vi "WaitBallTrajSkill.vi"(8 "error in (no error)":errorcluster, 9 "Robot":refnum<class "Robot.lvclass">, 10 "Game":refnum<class "Game.lvclass">, 11 "WaitBallTrajSkill in":refnum<class "WaitBallTrajSkill.lvclass">) -> (0 "error out":errorcluster, 2 "robot out":refnum<class "Robot.lvclass">, 3 "WaitBallTrajSkill out":refnum<class "WaitBallTrajSkill.lvclass">)   [LabVIEW 2023, in "WaitBallTrajSkill.lvclass"]
uses:
  WaitBallTrajSkill.lvclass
  Game_class/Game.lvclass
  Robot_class/Robot.lvclass
  Object_class/Object.lvclass/Object.ctl
  Game_class/Game.lvclass/Game.ctl
  Ball_class/Ball.lvclass/Ball.ctl
  Robot_class/Robot.lvclass/Robot.ctl
  Game_class/Read BallRef.vi
  Game_class/Read Utilities.lvclass.vi
  Game_class/Read FieldRef.vi
  Object_class/Read x.vi
  Object_class/Read y.vi
  Ball_class/Read v_x.vi
  Ball_class/Read v_y.vi
  Robot_class/Write dest_x.vi
  Robot_class/Write dest_y.vi
  Robot_class/Write dest_orientation.vi
  Ball_class/Ball.lvclass
  Utilities_class/Utilities.lvclass
  Field_class/Field.lvclass
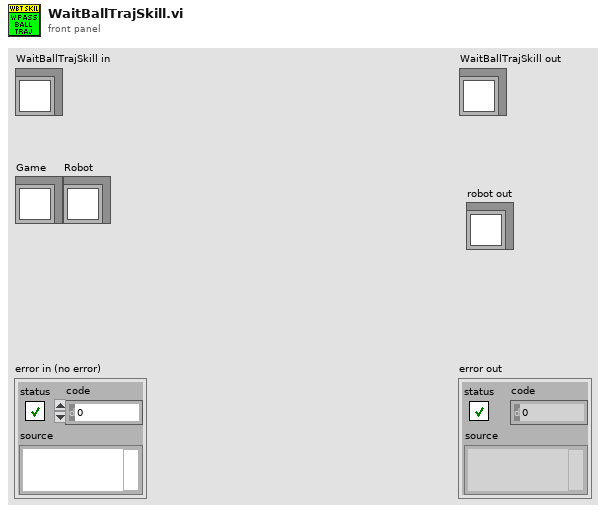
[diagram p1: front panel]
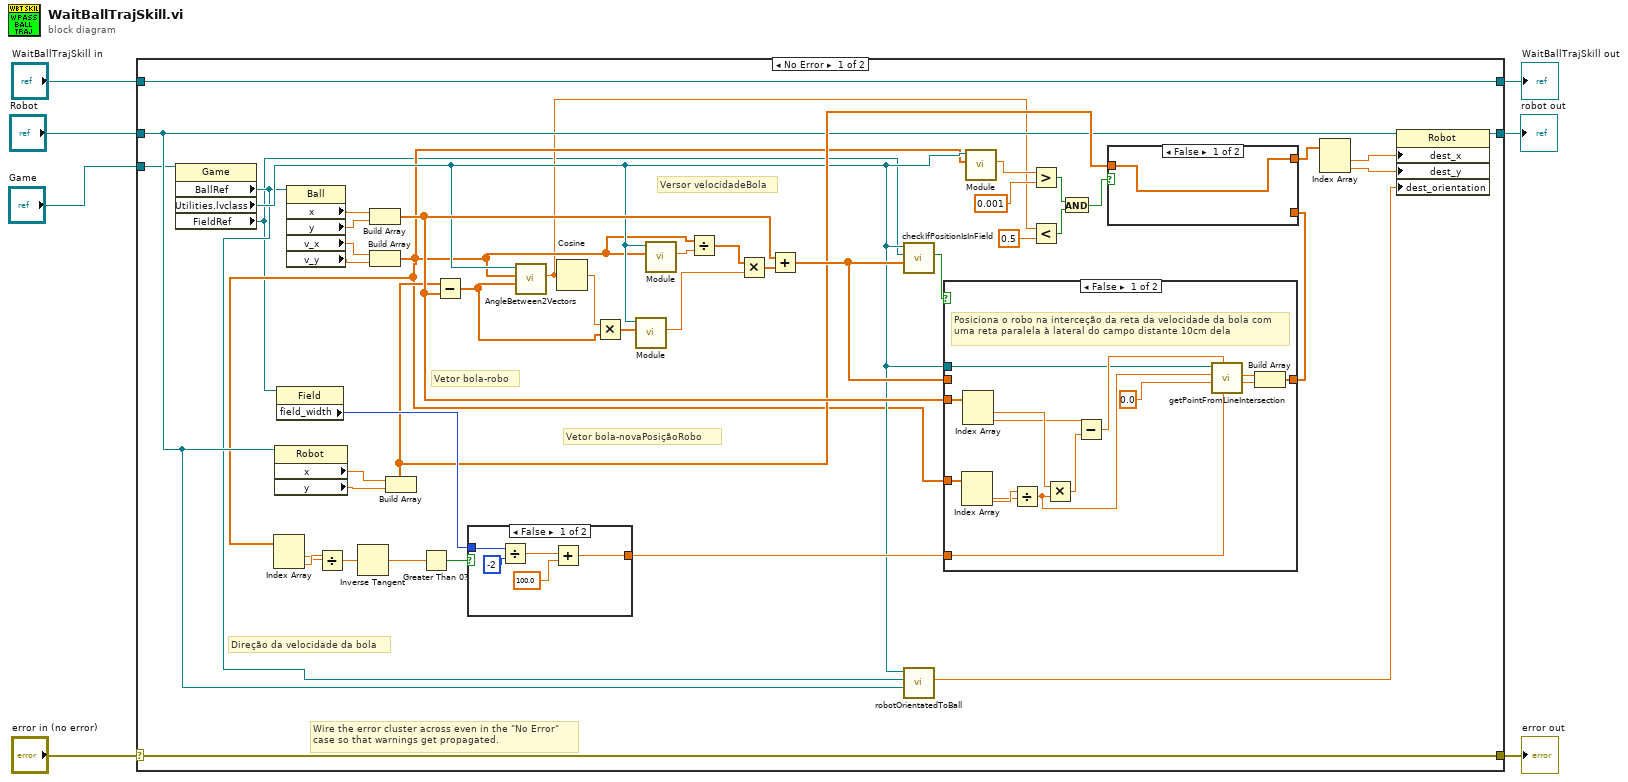
[diagram p0: block diagram]
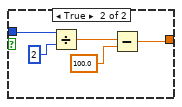
[diagram p3: hidden frame]
diagram:
  n1 = case shown="No Error" "error in (no error)" {
    selector: "error in (no error)" -> [w51 w82]
    tunnel: [w51 w82] -> w6
    tunnel: [w52 w81] -> w4
    tunnel: "WaitBallTrajSkill in" -> [w52 w81]
    tunnel: "Robot" -> [w23 _]
    tunnel: "Game" -> [w22 _]
    tunnel: [w50 _] -> w1
    frame No Error {
      # "Versor velocidadeBola"
      # "Direção da velocidade da bola"
      # "Vetor bola-novaPosiçãoRobo"
      # "Vetor bola-robo"
      # "Wire the error cluster across even in the \"No Error\"\ncase so that warnings get propagated."
      n2 = property class="Game"(reference=w22) -> ("BallRef"=w9:refnum<class "Ball.lvclass">, "Utilities.lvclass"=w20:refnum<class "Utilities.lvclass">, "FieldRef"=w8:refnum<class "Field.lvclass">)  [unwired: 1 in, 2 out]
      n3 = property class="Robot"(reference=w23) -> ("x"=w45:dbl, "y"=w44:dbl)  [unwired: 1 in, 2 out]
      n4 = property class="Field"(reference=w8) -> ("field_width"=w33:i32)  [unwired: 1 in, 2 out]
      n5 = property class="Ball"(reference=w9) -> ("x"=w49:dbl, "y"=w48:dbl, "v_x"=w46:dbl, "v_y"=w47:dbl)  [unwired: 1 in, 2 out]
      n6 = Build Array(w49, w48) -> (w31:dbl[])
      n7 = Build Array(w46, w47) -> (w18:dbl[])
      n8 = Index Array(array=w18) -> (element #1=w36:dbl, element #2=w37:dbl)  [unwired: 2 in]
      n9 = Divide(x=w37, y=w36) -> (x/y=w35:dbl)
      n10 = Inverse Tangent(1:w35) -> (0:w30:dbl)
      n11 = Build Array(w45, w44) -> (w25:dbl[])
      n12 = Greater Than 0?(x=w30) -> (x > 0?=w34:bool)
      n13 = Subtract(x=w25, y=w31) -> (x-y=w43:dbl[])
      n14 = case shown="False" w34 {
        tunnel: w33 -> [w58 w64]
        tunnel: [w57 w62] -> w32
        frame False {
          n15 = Divide(x=w58, y=-2) -> (x/y=w56:dbl)
          n16 = Add(x=w56, y=100.0) -> (x+y=w57:dbl)
        }
        frame True {
          n17 = Divide(x=w64, y=2) -> (x/y=w61:dbl)
          n18 = Subtract(x=w61, y=100.0) -> (x-y=w62:dbl)
        }
      }
      n19 = call "AngleBetween2Vectors.vi"("Array 1"=w43, "Array 2"=w18, "Utilities in"=w20) -> ("Numeric"=w10:dbl)  [unwired: 6 in, 2 out]
      n20 = Cosine(x=w10) -> (cos(x)=w42:dbl)
      n21 = Multiply(x=w42, y=w43) -> (x*y=w21:dbl[])
      n22 = call-dynamic "Module.vi"("2D vector"=w21, "Utilities in"=w20) -> ("Modulo"=w15:dbl)  [unwired: 7 in, 2 out]
      n23 = call-dynamic "Module.vi"("2D vector"=w18, "Utilities in"=w20) -> ("Modulo"=w19:dbl)  [unwired: 7 in, 2 out]
      n24 = Divide(x=w18, y=w19) -> (x/y=w16:dbl[])
      n25 = Multiply(x=w16, y=w15) -> (x*y=w17:dbl[])
      n26 = Add(x=w31, y=w17) -> (x+y=w40:dbl[])
      n27 = call "checkIfPositionIsInField.vi"("Position"=w40, "FieldRef"=w8, "Utilities in"=w20) -> ("Position Is In Field?"=w41:bool)  [unwired: 4 in, 4 out]
      n28 = call "robotOrientatedToBall.vi"("Robot"=w23, "BallRef"=w9, "Utilities in"=w20) -> ("Orientation"=w24:dbl)  [unwired: 6 in, 2 out]
      n29 = case shown="False" w41 {
        tunnel: w40 -> [_ w80]
        tunnel: [w77 w80] -> w29
        tunnel: w32 -> [w75 _]
        tunnel: w31 -> [w74 _]
        tunnel: w18 -> [w73 _]
        tunnel: w20 -> [w65 _]
        frame False {
          # "Posiciona o robo na interceção da reta da velocidade da bola com uma reta paralela à lateral do campo distante 10cm dela"
          n30 = Index Array(array=w73) -> (element #1=w71:dbl, element #2=w72:dbl)  [unwired: 2 in]
          n31 = Index Array(array=w74) -> (element #1=w70:dbl, element #2=w69:dbl)  [unwired: 2 in]
          n32 = Divide(x=w72, y=w71) -> (x/y=w66:dbl)
          n33 = Multiply(x=w70, y=w66) -> (x*y=w68:dbl)
          n34 = Subtract(x=w69, y=w68) -> (x-y=w67:dbl)
          n35 = call "getPointFromLineIntersection.vi"("b2"=w75, "b1"=w67, "a2"=0.0, "a1"=w66, "Utilities in"=w65) -> ("y_intersection"=w78:dbl, "x_intersection"=w79:dbl)  [unwired: 3 in, 2 out]
          n36 = Build Array(w79, w78) -> (w77:dbl[])
        }
        frame True {
        }
      }
      n37 = call-dynamic "Module.vi"("2D vector"=w18, "Utilities in"=w20) -> ("Modulo"=w27:dbl)  [unwired: 7 in, 2 out]
      n38 = Greater?(x=w27, y=0.001) -> (0:w12:bool)
      n39 = Less?(x=w10, y=0.5) -> (x < y?=w13:bool)
      n40 = And(x=w12, y=w13) -> (x .and. y?=w11:bool)
      n41 = case shown="False" w11 {
        tunnel: w29 -> [_ w54]
        tunnel: [w53 w54] -> w28
        tunnel: w25 -> [w53 _]
        frame False {
        }
        frame True {
        }
      }
      n42 = Index Array(array=w28) -> (element #1=w39:dbl, element #2=w38:dbl)  [unwired: 2 in]
      n43 = property class="Robot"(reference=w23, "dest_x"=w39, "dest_y"=w38, "dest_orientation"=w24) -> (reference out=w50:refnum<class "Robot.lvclass">)  [unwired: 1 in, 1 out]
    }
    frame Error {
    }
  }
  "error out" <- w6
  "WaitBallTrajSkill out" <- w4
  "robot out" <- w1
